vi "open file.vi"(8 "error in (no error)":errorcluster caption="에러 입력(에러 없음)", 10 "file path":path, 11 "WAV File 입력":refnum<class "WAV File.lvclass">) -> (0 "error out":errorcluster caption="에러 출력", 3 "WAV File 출력":refnum<class "WAV File.lvclass">)   [LabVIEW 2020, in "WAV File.lvclass"]
uses:
  WAV File.lvclass
  Waveform Obj/Waveform Obj.lvclass/Waveform Obj.ctl
  WAV File.lvclass/WAV File.ctl
  Waveform File/Waveform File.lvclass/Waveform File.ctl
  Waveform Obj/Accessors/Write name.vi
  Accessors/Write sound format.vi
  Waveform File/Accessors/Write source waveform.vi
  <vilib>/sound2/lvsound2.llb/Sound File Read Open.vi
  <vilib>/sound2/lvsound2.llb/Sound File Info (refnum).vi
  <vilib>/sound2/lvsound2.llb/Sound File Read (DBL).vi
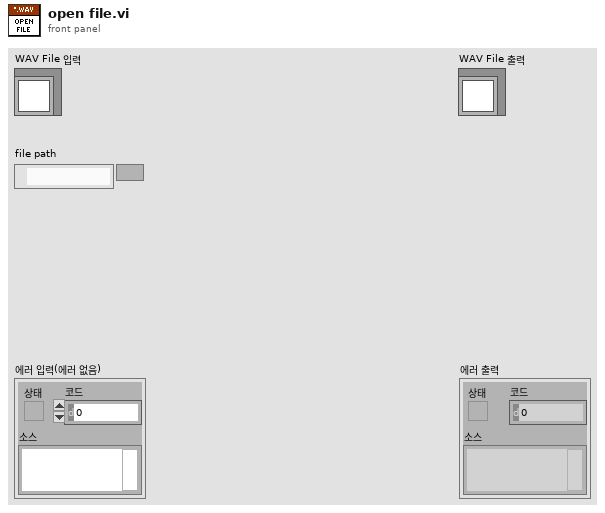
[diagram p1: front panel]
types:
  T1 = typedef "Sound File Refnum.ctl" = refnum<file>
  T2 = typedef "Sound Data Format.ctl" = cluster{"sample rate (S/s)":dbl, "number of channels":i32, "bits per sample":i32}
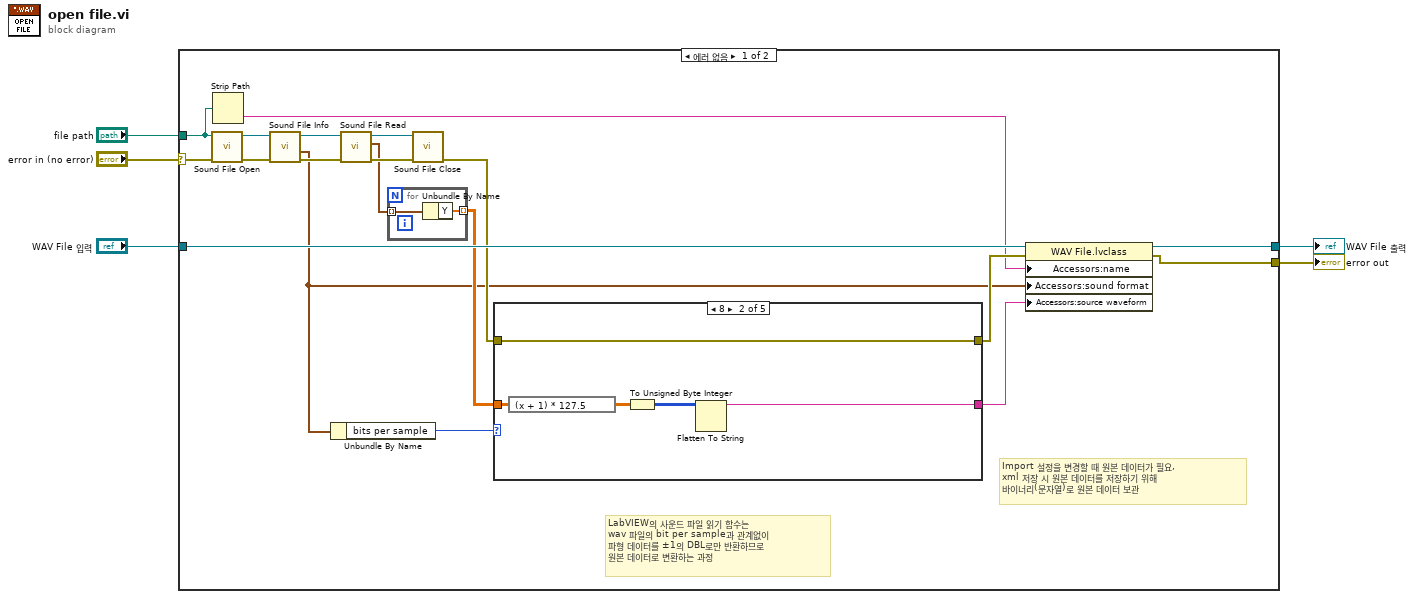
[diagram p0: block diagram]
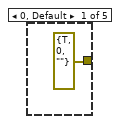
[diagram p2: hidden frame]
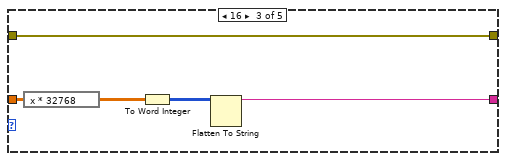
[diagram p3: hidden frame]
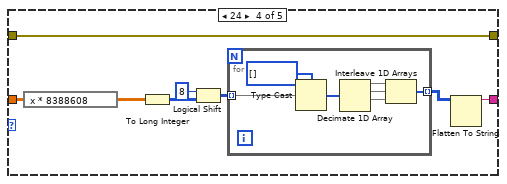
[diagram p4: hidden frame]
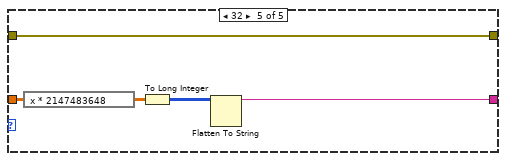
[diagram p5: hidden frame]
diagram:
  n1 = case shown="에러 없음" "error in (no error)" {
    selector: "error in (no error)" -> [w19 w58]
    tunnel: "WAV File 입력" -> [w22 w59]
    tunnel: [w21 w59] -> w3
    tunnel: [w20 w58] -> w2
    tunnel: "file path" -> [w7 _]
    frame No Error {
      # "Import 설정을 변경할 때 원본 데이터가 필요,\nxml 저장 시 원본 데이터를 저장하기 위해\n바이너리(문자열)로 원본 데이터 보관"
      # "LabVIEW의 사운드 파일 읽기 함수는 \nwav 파일의 bit per sample과 관계없이\n파형 데이터를 ±1의 DBL로만 반환하므로\n원본 데이터로 변환하는 과정"
      n2 = call-poly <vilib>:"Sound File Open.vi"("error in (no error)"=w19, "path"=w7) -> ("error out"=w17:errorcluster, "sound file refnum"=w18:T1)  [unwired: 8 in]
      n3 = Strip Path(path=w7) -> (name=w6:string)  [unwired: 1 out]
      n4 = call-poly <vilib>:"Sound File Info.vi"("error in (no error)"=w17, "sound file refnum"=w18) -> ("error out"=w15:errorcluster, "sound format"=w8:T2, "sound file refnum out"=w16:T1)  [unwired: 6 in, 1 out]
      n5 = Unbundle By Name(w8) -> ("bits per sample"=w14:i32)
      n6 = call-poly <vilib>:"Sound File Read.vi"("error in (no error)"=w15, "sound file refnum"=w16) -> ("error out"=w23:errorcluster, "data"=w13:waveform(dbl)[], "sound file refnum out"=w24:T1)  [unwired: 5 in, 2 out]
      n7 = for {
        tunnel: w13 -> [w26] mode=indexing
        tunnel: [w25] -> w12 mode=indexing
        n8 = Unbundle By Name(w26) -> ("Y"=w25:dbl[])
      }
      n9 = call <vilib>:"Sound File Close.vi"("error in (no error)"=w23, "sound file refnum"=w24) -> ("error out"=w10:errorcluster)  [unwired: 9 in]
      n10 = case shown="8" w14 {
        tunnel: w12 -> [_ w32 w37 w45 w57]
        tunnel: [_ w29 w34 w43 w54] -> w11
        tunnel: w10 -> [_ w28 w33 w38 w53]
        tunnel: [errorcluster {"status"=TRUE, "code"=0, "source"=""} ("error out") w28 w33 w38 w53] -> w9
        frame 0, Default {
        }
        frame 8 {
          n11 = expression code="(x + 1) * 127.5"(w32) -> (w31:dbl[][])
          n12 = To Unsigned Byte Integer(number=w31) -> (unsigned 8bit integer=w30:u8[][])
          n13 = Flatten To String(anything=w30) -> (data string=w29:string)  [unwired: 3 in, 2 out]
        }
        frame 16 {
          n14 = expression code="x * 32768"(w37) -> (w36:dbl[][])
          n15 = To Word Integer(number=w36) -> (16bit integer=w35:i16[][])
          n16 = Flatten To String(anything=w35) -> (data string=w34:string)  [unwired: 3 in, 2 out]
        }
        frame 24 {
          n17 = expression code="x * 8388608"(w45) -> (w44:dbl[][])
          n18 = To Long Integer(number=w44) -> (32bit integer=w42:i32[][])
          n19 = Logical Shift(y=i16 8, x=w42) -> (x << y=w41:i32[][])
          n20 = for {
            tunnel: w41 -> [w52] mode=indexing
            tunnel: [w46] -> w39 mode=indexing
            n21 = Type Cast(type=u8[] [], x=w52) -> (*(type *) &x=w50:u8[])
            n22 = Decimate 1D Array(w50) -> (w49:u8[], w48:u8[], w47:u8[])  [unwired: 1 out]
            n23 = Interleave 1D Arrays(w49, w48, w47) -> (w46:u8[])
          }
          n24 = Flatten To String(anything=w39) -> (data string=w43:string)  [unwired: 3 in, 2 out]
        }
        frame 32 {
          n25 = expression code="x * 2147483648"(w57) -> (w56:dbl[][])
          n26 = To Long Integer(number=w56) -> (32bit integer=w55:i32[][])
          n27 = Flatten To String(anything=w55) -> (data string=w54:string)  [unwired: 3 in, 2 out]
        }
      }
      n28 = property class="WAV File.lvclass"(reference=w22, error in=w9, "Accessors:name"=w6, "Accessors:sound format"=w8, "Accessors:source waveform"=w11) -> (reference out=w21:refnum<class "WAV File.lvclass">, error out=w20:errorcluster)
    }
    frame Error {
    }
  }
  "error out" <- w2
  "WAV File 출력" <- w3
